vi "rsp_Timeout.vi"(4 "Show in Debugger?":bool=TRUE, 6 "Message Priority":T1=enum."Normal", 8 "error in":errorcluster, 10 "Data in":T2={"Data"=variant(string ""), "Auxiliary"=variant}, 11 "Work Planer in":refnum<class "Work Planer.lvclass">) -> (0 "error out":errorcluster, 3 "dup Work Planer out":refnum<class "Work Planer.lvclass">)   [LabVIEW 2023, in "Work Planer.lvclass"]
doc: "This VI sends a <b>Public API Response</b> message to a registered MHL case of the Caller of the Worker that owns this VI.\n---\nЗаданное время прошло, отправляем caller'у"
uses:
  Work Planer.lvclass
  rsp_Timeout.ctl
  <vilib>/addons/_Workers/Library/Classes/Message/Priority.ctl
  Work Planer.lvclass/Work Planer.ctl
  <vilib>/Utility/error.llb/Error Cluster From Error Code.vi
  <vilib>/addons/_Workers/Library/Classes/Worker/Worker.lvclass
  <vilib>/addons/_Workers/Library/Classes/Message Queue/Message Queue.lvclass
  <vilib>/ErrorRing/Error Ring.xnode
  <vilib>/addons/_Workers/Library/Classes/Message/Message.lvclass
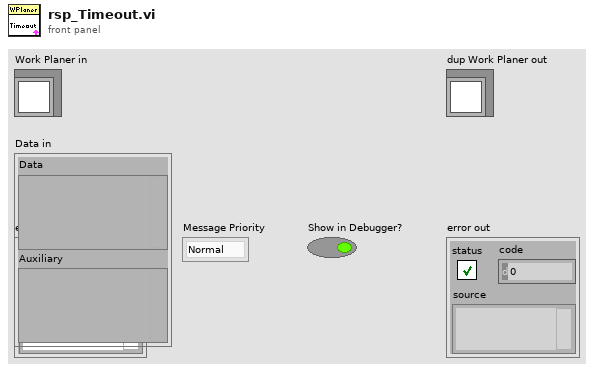
[diagram p1: front panel]
types:
  T1 = typedef "Workers.lvlib/Message.lvclass/Priority.ctl" = enum16{"Low", "Normal", "High"}
  T2 = typedef "Work Planer.lvclass/rsp_Timeout.ctl" = cluster{"Data":variant, "Auxiliary":variant}
  T3 = typedef "Workers.lvlib/Case Label.ctl" = string
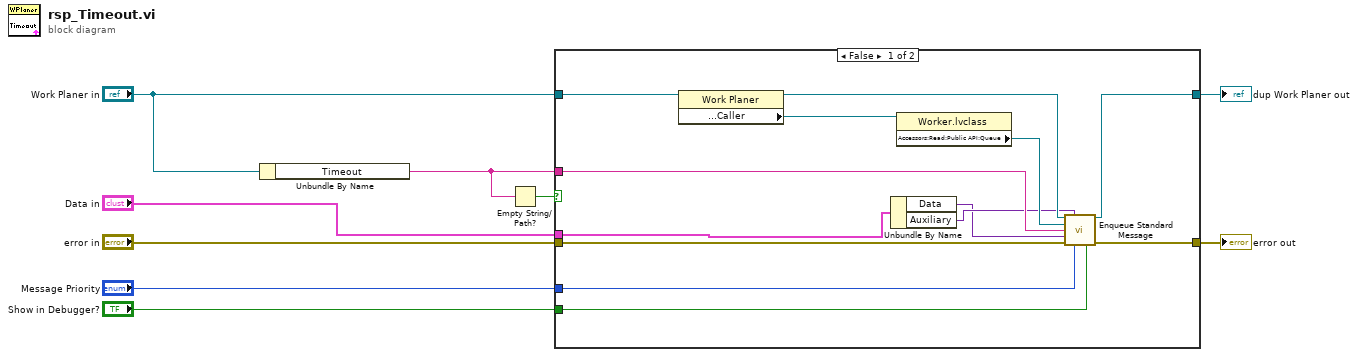
[diagram p0: block diagram]
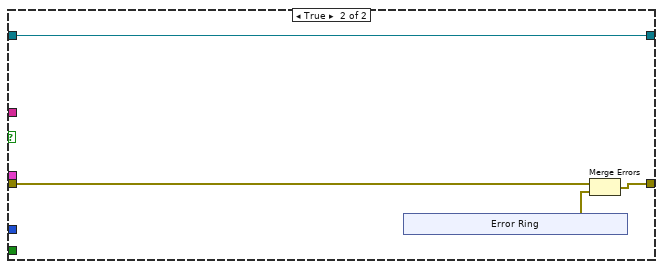
[diagram p2: hidden frame]
diagram:
  n1 = Unbundle By Name("Work Planer in") -> ("Timeout"=w4:T3)
  n2 = Empty String/Path?(string/path=w4) -> (empty?=w5:bool)
  n3 = case shown="False" w5 {
    tunnel: "error in" -> [w22 w23]
    tunnel: [w21 w24] -> w8
    tunnel: "Data in" -> [w12 _]
    tunnel: [w20 w26] -> w6
    tunnel: "Work Planer in" -> [w16 w26]
    tunnel: w4 -> [w19 _]
    tunnel: "Show in Debugger?" -> [w18 _]
    tunnel: "Message Priority" -> [w17 _]
    frame False {
      n4 = property class="Work Planer"(reference=w16) -> (reference out=w15:refnum<class "Work Planer.lvclass">, "Accessors:Read:Public API:Caller"=w13:refnum<class "Worker.lvclass">)  [unwired: 1 in, 1 out]
      n5 = Unbundle By Name(w12) -> ("Data"=w10:variant, "Auxiliary"=w11:variant)
      n6 = property class="Worker.lvclass"(reference=w13) -> ("Accessors:Read:Public API:Queue"=w14:refnum<class "Message Queue.lvclass">)  [unwired: 1 in, 2 out]
      n7 = call-dynamic "Enqueue Standard Message.vi"("Worker"=w15, "Auxiliary"=w11, "Message Queue"=w14, "Case Label"=w19, "Data"=w10, "error in (no error)"=w22, "Priority (Normal)"=w17, "Send Message to Debugger? (T)"=w18) -> ("dup Worker out"=w20:refnum<class "Work Planer.lvclass">, "error out"=w21:errorcluster)  [unwired: 6 in]
    }
    frame True {
      n8 = xnode "Error Ring"() -> ("error out"=w25:errorcluster)
      n9 = Merge Errors(w23, w25) -> (w24:errorcluster)
    }
  }
  "error out" <- w8
  "dup Work Planer out" <- w6
